vi "Harmonics MSMT Set RF WFM Parameters.vi"(8 "error in (no error)":errorcluster, 10 "Step In":refnum<k7>, 11 "Harmonics in":refnum<class "Harmonics.lvclass">) -> (0 "error out":errorcluster, 2 "Step Out":refnum<k7>, 3 "Harmonics MSMT out":refnum<class "Harmonics.lvclass">)   [LabVIEW 2018, in "Harmonics.lvlib" / "Harmonics.lvclass"]
uses:
  Harmonics.lvclass
  C:/Sequence Automation/Plugins/Measurement Interface.lvlibp/Measurement Interface.lvclass
  Plugins/Measurement Interface.lvlibp/Private Methods/Measurement Parameters/Read Measurement Parameters.vi
  Plugins/String Database.lvlibp/String Database.lvclass
  Plugins/TestStand API Tools (TSAT).lvlibp/Step Actions/TSAT Step Actions.lvlib
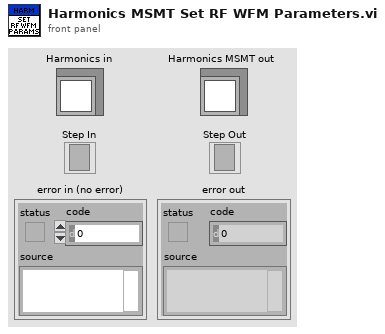
[diagram p1: front panel]
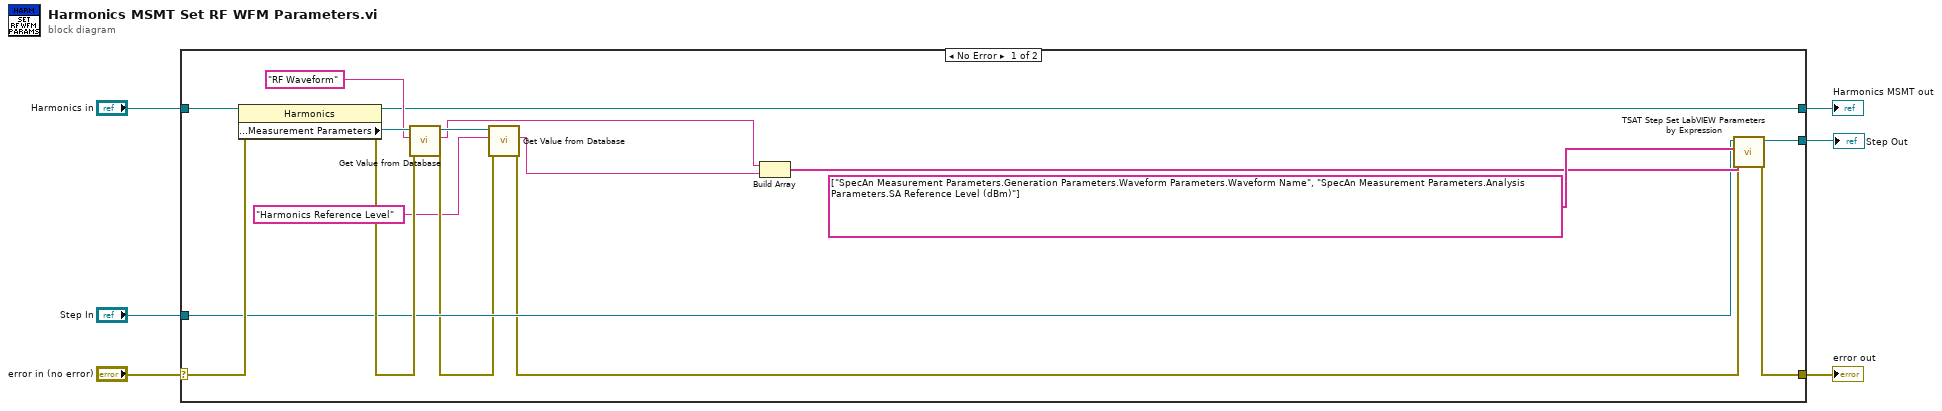
[diagram p0: block diagram]
diagram:
  n1 = case shown="No Error" "error in (no error)" {
    selector: "error in (no error)" -> [w23 w26]
    tunnel: [w22 w26] -> w5
    tunnel: [w8 w25] -> w3
    tunnel: "Harmonics in" -> [w21 w25]
    tunnel: [w15 w24] -> w2
    tunnel: "Step In" -> [w14 w24]
    frame No Error {
      n2 = property class="Harmonics"(reference=w21, error in=w23) -> (reference out=w8:refnum<class "Harmonics.lvclass">, error out=w19:errorcluster, "Protected Methods:Measurement Parameters"=w20:refnum<class "String Database.lvclass">)
      n3 = call "Get Value from Database.vi"("error in (no error)"=w19, "Entry Name"="RF Waveform", "Message in"=w20) -> ("error out"=w12:errorcluster, "Entry Value"=w7:string, "Message out"=w13:refnum<class "String Database.lvclass">)  [unwired: 5 in, 1 out]
      n4 = call "Get Value from Database.vi"("error in (no error)"=w12, "Entry Name"="Harmonics Reference Level", "Message in"=w13) -> ("error out"=w11:errorcluster, "Entry Value"=w9:string)  [unwired: 5 in, 2 out]
      n5 = Build Array(w7, w9) -> (w16:string[])
      n6 = call "TSAT Step Set LabVIEW Parameters by Expression.vi"("Error In"=w11, "Value Expressions"=w16, "Parameters to Set"=string[] ["SpecAn Measurement Parameters.Generation Parameters.Waveform Parameters.Waveform Name", "SpecAn Measurement Parameters.Analysis Parameters.SA Reference Level (dBm)"], "Step In"=w14) -> ("Error Out"=w22:errorcluster, "Step Out"=w15:refnum<k7>)  [unwired: 6 in]
    }
    frame Error {
    }
  }
  "error out" <- w5
  "Harmonics MSMT out" <- w3
  "Step Out" <- w2
